vi "Read Level Occurrence Time.vi"(5 "Pulse Width (0)":dbl, 6 "Start Time (0.005)":dbl=0.005, 7 "Absolute Level (100)":dbl=100.0, 8 "error in (no error)":errorcluster, 9 "Occurrence (-1)":dbl=-1.0, 10 "Level (10)":dbl=10.0, 11 "VISA resource name":refnum<visa-resource-name>) -> (0 "error out":errorcluster, 1 "Absolute Time":dbl, 2 "Time":dbl, 3 "VISA resource name out":refnum<visa-resource-name>)   [LabVIEW 2020, in "Agilent 681x Series.lvlib"]
doc: "Returns the time at which the measured voltage and absolute value of the measured voltage crosses a user-specified voltage level."
uses:
  <instrlib>/Agilent 681x Series/Agilent 681x Series.lvlib
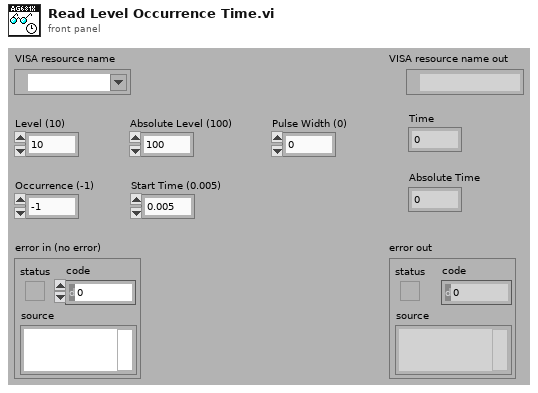
[diagram p1: front panel]
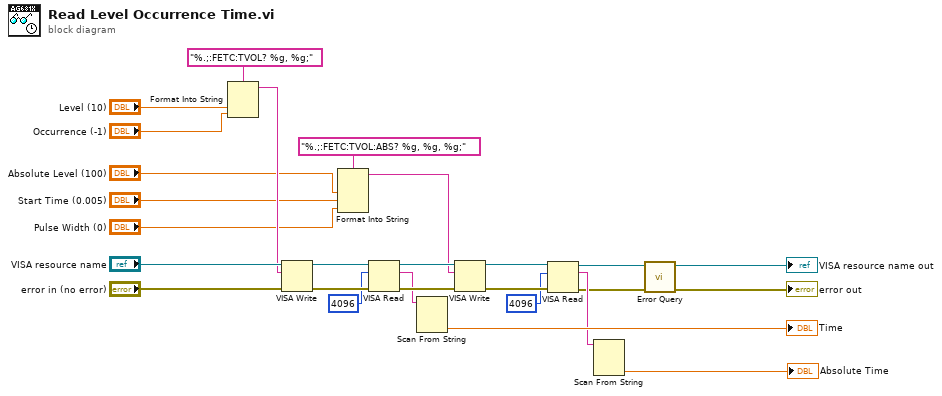
[diagram p0: block diagram]
diagram:
  n1 = Format Into String(format string="%.;:FETC:TVOL? %g, %g;", "Level (10)", "Occurrence (-1)") -> (resulting string=w19:string)  [unwired: 2 in, 1 out]
  n2 = VISA Write(VISA resource name="VISA resource name", write buffer=w19, error in (no error)="error in (no error)") -> (VISA resource name out=w23:refnum<visa-resource-name>, error out=w22:errorcluster)  [unwired: 1 out]
  n3 = Format Into String(format string="%.;:FETC:TVOL:ABS? %g, %g, %g;", "Absolute Level (100)", "Start Time (0.005)", "Pulse Width (0)") -> (resulting string=w9:string)  [unwired: 2 in, 1 out]
  n4 = VISA Read(VISA resource name=w23, byte count=u32 4096, error in (no error)=w22) -> (VISA resource name out=w14:refnum<visa-resource-name>, read buffer=w5:string, error out=w13:errorcluster)  [unwired: 1 out]
  n5 = Scan From String(input string=w5) -> (output 1=→"Time":dbl)  [unwired: 4 in, 3 out]
  n6 = VISA Write(VISA resource name=w14, write buffer=w9, error in (no error)=w13) -> (VISA resource name out=w12:refnum<visa-resource-name>, error out=w11:errorcluster)  [unwired: 1 out]
  n7 = VISA Read(VISA resource name=w12, byte count=u32 4096, error in (no error)=w11) -> (VISA resource name out=w4:refnum<visa-resource-name>, read buffer=w6:string, error out=w2:errorcluster)  [unwired: 1 out]
  n8 = Scan From String(input string=w6) -> (output 1=→"Absolute Time":dbl)  [unwired: 4 in, 3 out]
  n9 = call <instrlib>:"Error Query.vi"("error in (no error)"=w2, "VISA resource name"=w4) -> ("error out"=→"error out":errorcluster, "VISA resource name out"=→"VISA resource name out":refnum<visa-resource-name>)  [unwired: 6 in, 2 out]
